vi "BT Example 9 - Queue Synch.vi"() -> ()   [LabVIEW 2021]
uses:
  Support/Nodes/abs_Node/Status.ctl
  System/bt_System.lvclass
  Support/Nodes/Composites/abs_Parallel/Support/Status Calculation.ctl
  Blackboard/Blackboard.lvclass
  Support/Nodes/Decorators/Repeater/Support/Finish On - Type.ctl
  Support/Synch Type 1.ctl
  Blackboard/Blackboard.lvclass/Blackboard.ctl
  Support/Nodes/Leaves/abs_Type Leaf/abs_Type Leaf.lvclass/abs_Type Leaf.ctl
  Blackboard/Get Value Type/Get I32.vi
  Blackboard/Support/Index Group.vi
  Blackboard/Support/Index Tags.vi
  Support/Nodes/Leaves/abs_Type Leaf/Properties/Write Value Class.vi
  <vilib>/TSA/Omni-Bus/Local Bus/Support/I32/Local Bus_I32.lvclass
  C:/Program Files (x86)/National Instruments/LabVIEW 2021/vi.lib/TSA/Abstract Data Classes/Abs_Types/Value/Abs_Value.lvclass
  <vilib>/TSA/Abstract Data Classes/Abs_Types/I32 Integer/Abs_I32 Integer.lvclass
  C:/Program Files (x86)/National Instruments/LabVIEW 2021/vi.lib/TSA/Abstract Data Classes/Abs_Types/Numeric/Abs_Numeric.lvclass
  Support/Nodes/Leaves/Test Boolean/Test Abs_Boolean.lvclass
  C:/Users/Tim/Documents/GitHub/LV_Behaviour_Tree/Source/Support/Nodes/abs_Node/bt_Node.lvclass
  C:/Users/Tim/Documents/GitHub/LV_Behaviour_Tree/Source/Support/Nodes/Leaves/abs_Type Leaf/abs_Type Leaf.lvclass
  <vilib>/TSA/Abstract Data Classes/Abs_Types/Boolean/Abs_Boolean.lvclass
  C:/Program Files (x86)/National Instruments/LabVIEW 2021/vi.lib/TSA/Abstract Data Classes/Abs_Types/Type/Abs_Type.lvclass
  <vilib>/TSA/Omni-Bus/Local Bus/Support/Initialise DVR's.vi
  <vilib>/TSA/Abstract Data Classes/Functions/Math/Support/Increment/I32/Method.vi
  <vilib>/TSA/Abstract Data Classes/Constants/Support/I32/I32.vi
  <vilib>/TSA/Abstract Data Classes/Functions/Compare/Support/Greater Equal/I32/Method.vi
  <vilib>/TSA/Abstract Data Classes/Abs_Types/Value/Abs_Value.lvclass
  <vilib>/TSA/Abstract Data Classes/Abs_Types/Type/Abs_Type.lvclass
  <vilib>/TSA/Omni-Bus/Local Bus/Support/DBL/Local Bus_DBL.lvclass
  <vilib>/TSA/Omni-Bus/Local Bus/Support/SGL/Local Bus_SGL.lvclass
  <vilib>/TSA/Omni-Bus/Local Bus/Support/EXT/Local Bus_EXT.lvclass
  <vilib>/TSA/Omni-Bus/Local Bus/Support/Bool/Local Bus_Boolean.lvclass
  <vilib>/TSA/Omni-Bus/Local Bus/Support/STR/Local Bus_String.lvclass
  <vilib>/TSA/Omni-Bus/Local Bus/Support/Variant/Local Bus_Variant.lvclass
  <vilib>/TSA/Omni-Bus/Local Bus/Support/WFM/Local Bus_Waveform.lvclass
  <vilib>/TSA/Omni-Bus/Local Bus/Support/Time/Local Bus_Time.lvclass
  <vilib>/TSA/Omni-Bus/Local Bus/Support/U8/Local Bus_U8.lvclass
  <vilib>/TSA/Omni-Bus/Local Bus/Support/U16/Local Bus_U16.lvclass
  <vilib>/TSA/Omni-Bus/Local Bus/Support/U32/Local Bus_U32.lvclass
  <vilib>/TSA/Omni-Bus/Local Bus/Support/U64/Local Bus_U64.lvclass
  <vilib>/TSA/Omni-Bus/Local Bus/Support/I8/Local Bus_I8.lvclass
  <vilib>/TSA/Omni-Bus/Local Bus/Support/I16/Local Bus_I16.lvclass
  <vilib>/TSA/Omni-Bus/Local Bus/Support/I64/Local Bus_I64.lvclass
  <vilib>/TSA/Omni-Bus/Local Bus/Support/CSGL/Local Bus_CSGL.lvclass
  <vilib>/TSA/Omni-Bus/Local Bus/Support/CDBL/Local Bus_CDBL.lvclass
  <vilib>/TSA/Omni-Bus/Local Bus/Support/CEXT/Local Bus_CEXT.lvclass
  <vilib>/TSA/Omni-Bus/Local Bus/Support/Type/Local Bus_Type.lvclass
  BT.lvlib
  Support/Nodes/Composites/abs_Parallel/bt_Parallel.lvclass
  Support/Nodes/Decorators/Repeater/bt_Repeater.lvclass
  C:/Program Files (x86)/National Instruments/LabVIEW 2021/vi.lib/TSA/Abstract Data Classes/Abs_Types/Integer/Abs_Integer.lvclass
  C:/Program Files (x86)/National Instruments/LabVIEW 2021/vi.lib/TSA/Abstract Data Classes/Abs_Types/I32 Integer/Abs_I32 Integer.lvclass
  <vilib>/TSA/Abstract Data Classes/Constants/Support/I32/Const_I32.lvclass
  <vilib>/TSA/Abstract Data Classes/Functions/Compare/Support/Greater Equal/I32/Greater Equal_I32.lvclass
  <vilib>/TSA/Abstract Data Classes/Functions/Math/Support/Increment/I32/Increment_I32.lvclass
  Support/Nodes/abs_Node/bt_Node.lvclass
panel:
  out "Tags Table":string[][](table)
  out "error out":errorcluster
  in  "stop":bool
  out "Status":T1
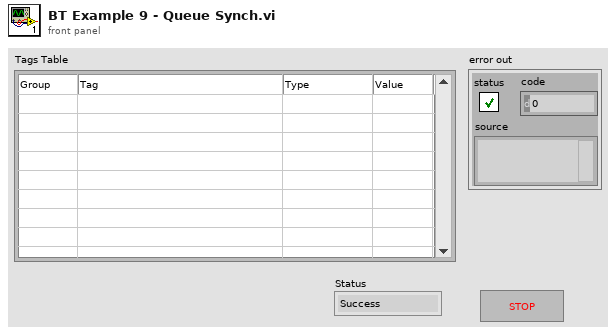
[diagram p1: front panel]
types:
  T1 = typedef "BT.lvlib/bt_Node.lvclass/Status.ctl" = enum16{"Success", "Failure", "Running"}
  T2 = typedef "Synch Type 1.ctl" = cluster{"n":i32, "Bool":bool, "Str":string, "Cluster":cluster{"Numeric":dbl, "Waveform":waveform(dbl), "Time Stamp":timestamp, "Variant":variant}}
  T3 = typedef "BT.lvlib/bt_Repeater.lvclass/Finish On - Type.ctl" = enum16{"Success", "Failure", "Never"}
  T4 = typedef "BT.lvlib/bt_Parallel.lvclass/Status Calculation.ctl" = enum16{"Succeed on All Succeed", "Failure on All Failure", "Succeed on Any Succeed", "Failure on Any Failure"}
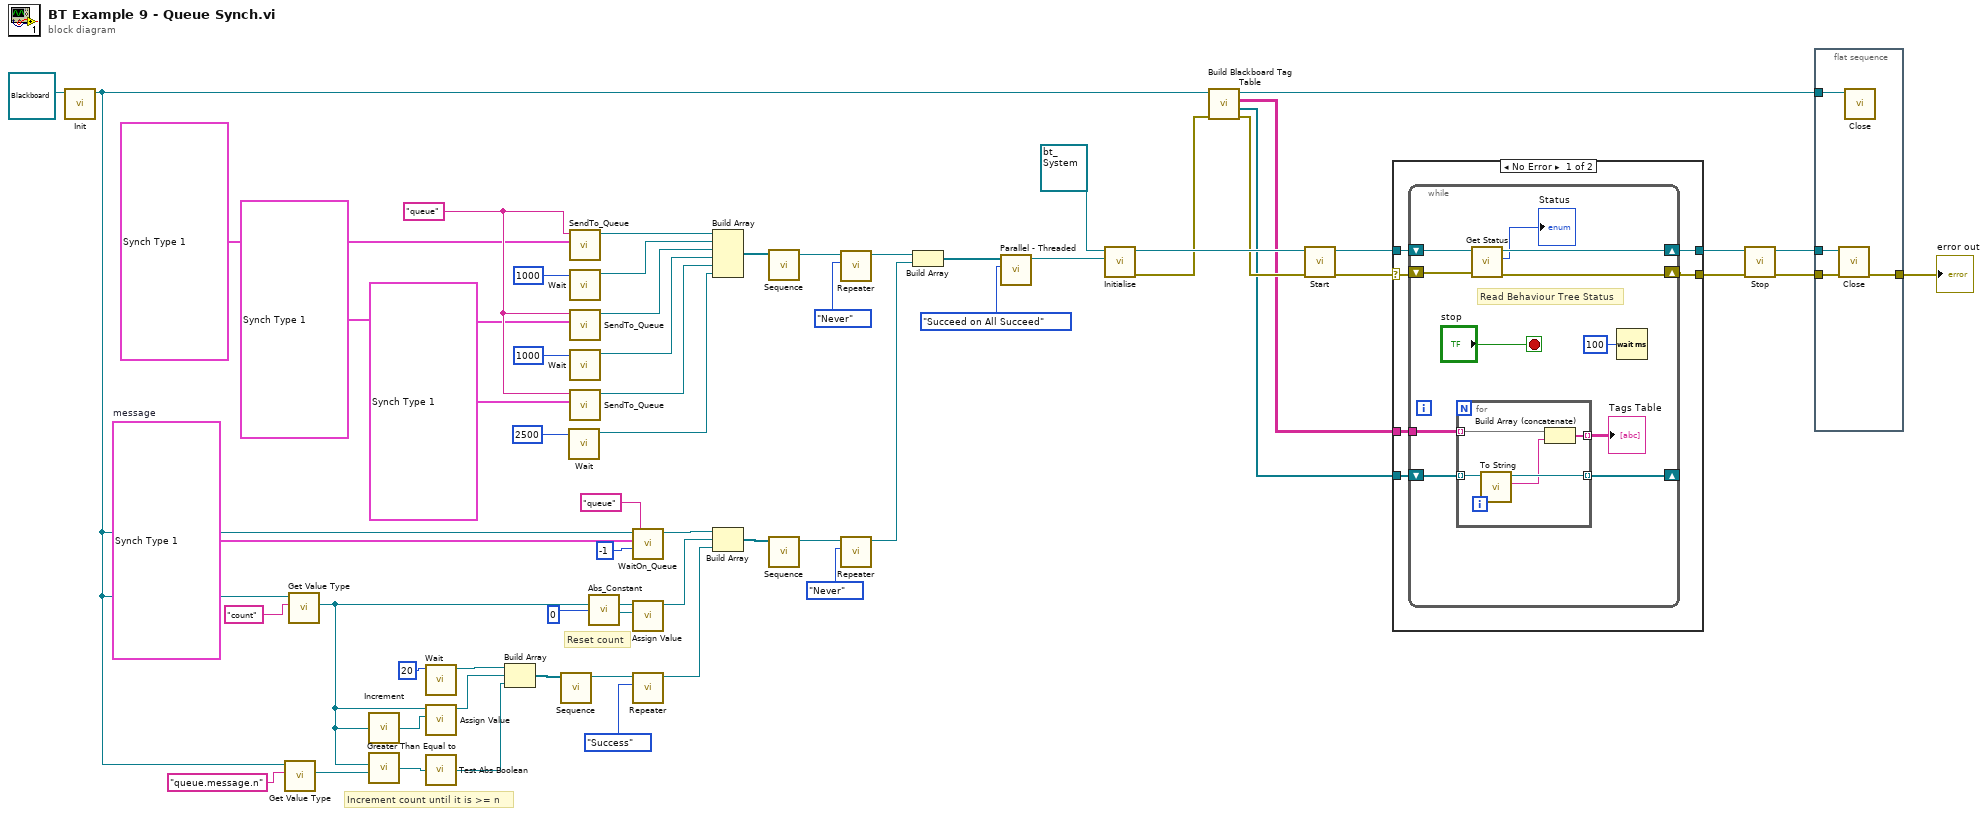
[diagram p0: block diagram]
diagram:
  w4 = T2 {"n"=0, "Bool"=TRUE, "Str"="", "Cluster"={"Numeric"=0.0, "Waveform"={"t0"=timestamp(0 s since 1904-01-01), "dt"=4.0, "Y"=[]}, "Time Stamp"=timestamp(0 s since 1904-01-01), "Variant"=variant}}  # message
  w10 = "queue" ("Name")
  # "Increment count until it is >= n"
  # "Reset count"
  n1 = call-dynamic "Init.vi"("bt_Blackboard in"=refnum<class "Blackboard.lvclass"> refnum) -> ("bt_Blackboard out"=w21:refnum<class "Blackboard.lvclass">)  [unwired: 9 in, 1 out]
  n2 = call-poly "Get Value Type.vi"("Tag"="queue.message.n", "Blackboard in"=w21) -> ("Value"=w22:refnum<class "Abs_I32 Integer.lvclass">)  [unwired: 6 in, 3 out]
  n3 = call-poly "Get Value Type.vi"("Tag"="count", "Blackboard in"=w21) -> ("Value"=w23:refnum<class "Abs_I32 Integer.lvclass">)  [unwired: 6 in, 3 out]
  n4 = call-poly <vilib>:"Increment.vi"("Value"=w23) -> ("Result"=w37:refnum<class "Abs_I32 Integer.lvclass">)  [unwired: 4 in]
  n5 = call-poly <vilib>:"Greater Than Equal to.vi"("Value B"=w22, "Value A"=w23) -> ("Result"=w35:refnum<class "Abs_Boolean.lvclass">)  [unwired: 4 in]
  n6 = call "Wait.vi"("Time (ms)"=u32 20) -> ("Node Out"=w32:refnum<class "bt_Node.lvclass">)  [unwired: 10 in]
  n7 = call "Assign Value.vi"("Assigned Value"=w37, "Value"=w23) -> ("Node Out"=w36:refnum<class "bt_Node.lvclass">)  [unwired: 9 in]
  n8 = call "Test Abs Boolean.vi"("Abs_Boolean.lvclass"=w35) -> ("abs_Node"=w34:refnum<class "bt_Node.lvclass">)  [unwired: 4 in]
  n9 = Build Array(w32, w36, w34) -> (w42:refnum<class "bt_Node.lvclass">[])
  n10 = call "Sequence.vi"("Nodes"=w42) -> ("Node"=w43:refnum<class "bt_Node.lvclass">)  [unwired: 10 in]
  n11 = call "Wait.vi"("Time (ms)"=u32 2500) -> ("Node Out"=w5:refnum<class "bt_Node.lvclass">)  [unwired: 10 in]
  n12 = call "SendTo_Queue.vi"("Message"=T2 {"n"=10, "Bool"=TRUE, "Str"="A", "Cluster"={"Numeric"=0.0, "Waveform"={"t0"=timestamp(0 s since 1904-01-01), "dt"=1.0, "Y"=[]}, "Time Stamp"=timestamp(0 s since 1904-01-01), "Variant"=variant}} ("message"), "Queue Name"=w10) -> ("Node Out"=w18:refnum<class "bt_Node.lvclass">)  [unwired: 9 in]
  n13 = call "Wait.vi"("Time (ms)"=u32 1000) -> ("Node Out"=w13:refnum<class "bt_Node.lvclass">)  [unwired: 10 in]
  n14 = call "SendTo_Queue.vi"("Message"=T2 {"n"=33, "Bool"=FALSE, "Str"="B", "Cluster"={"Numeric"=0.0, "Waveform"={"t0"=timestamp(0 s since 1904-01-01), "dt"=2.0, "Y"=[]}, "Time Stamp"=timestamp(0 s since 1904-01-01), "Variant"=variant}} ("data"), "Queue Name"=w10) -> ("Node Out"=w16:refnum<class "bt_Node.lvclass">)  [unwired: 9 in]
  n15 = call "Wait.vi"("Time (ms)"=u32 1000) -> ("Node Out"=w11:refnum<class "bt_Node.lvclass">)  [unwired: 10 in]
  n16 = call "SendTo_Queue.vi"("Message"=T2 {"n"=100, "Bool"=TRUE, "Str"="C", "Cluster"={"Numeric"=0.0, "Waveform"={"t0"=timestamp(0 s since 1904-01-01), "dt"=3.0, "Y"=[]}, "Time Stamp"=timestamp(0 s since 1904-01-01), "Variant"=variant}} ("data"), "Queue Name"=w10) -> ("Node Out"=w15:refnum<class "bt_Node.lvclass">)  [unwired: 9 in]
  n17 = call-poly <vilib>:"Abs_Constant.vi"("Value"=0 ("n")) -> ("Constant"=w38:refnum<class "Abs_I32 Integer.lvclass">)  [unwired: 4 in]
  n18 = call "WaitOn_Queue.vi"("Queue Name"="queue" ("Name"), "Timeout (ms)"=-1, "Message Type"=w4, "bt_Blackboard in"=w21) -> ("Node Out"=w24:refnum<class "bt_Node.lvclass">)  [unwired: 6 in, 1 out]
  n19 = call "Assign Value.vi"("Assigned Value"=w38, "Value"=w23) -> ("Node Out"=w33:refnum<class "bt_Node.lvclass">)  [unwired: 9 in]
  n20 = call "Repeater.vi"("Finish On"=Finish_On_-_Type."Success", "Node In"=w43) -> ("Node Out"=w44:refnum<class "bt_Node.lvclass">)  [unwired: 9 in]
  n21 = Build Array(w18, w13, w16, w11, w15, w5) -> (w17:refnum<class "bt_Node.lvclass">[])
  n22 = Build Array(w24, w33, w44) -> (w46:refnum<class "bt_Node.lvclass">[])
  n23 = call "Sequence.vi"("Nodes"=w17) -> ("Node"=w8:refnum<class "bt_Node.lvclass">)  [unwired: 10 in]
  n24 = call "Sequence.vi"("Nodes"=w46) -> ("Node"=w45:refnum<class "bt_Node.lvclass">)  [unwired: 10 in]
  n25 = call "Repeater.vi"("Finish On"=Finish_On_-_Type."Never", "Node In"=w8) -> ("Node Out"=w7:refnum<class "bt_Node.lvclass">)  [unwired: 9 in]
  n26 = call "Repeater.vi"("Finish On"=Finish_On_-_Type."Never", "Node In"=w45) -> ("Node Out"=w52:refnum<class "bt_Node.lvclass">)  [unwired: 9 in]
  n27 = Build Array(w7, w52) -> (w55:refnum<class "bt_Node.lvclass">[])
  n28 = call "Parallel - Threaded.vi"("Status Calculation"=Status_Calculation."Succeed on All Succeed", "Nodes"=w55) -> ("Node"=w54:refnum<class "bt_Node.lvclass">)  [unwired: 9 in]
  n29 = call "Initialise.vi"("Behaviour Tree"=w54, "bt_System in"=refnum<class "bt_System.lvclass"> refnum) -> ("error out"=w25:errorcluster, "bt_System out"=w28:refnum<class "bt_System.lvclass">)  [unwired: 8 in]
  n30 = call "Build Blackboard Tag Table.vi"("error in (no error)"=w25, "Blackboard in"=w21) -> ("error out"=w27:errorcluster, "Values"=w20:refnum<class "Abs_Value.lvclass">[], "Table"=w19:string[][], "Blackboard out"=w26:refnum<class "Blackboard.lvclass">)  [unwired: 6 in]
  n31 = call "Start.vi"("error in (no error)"=w27, "bt_System in"=w28) -> ("error out"=w49:errorcluster, "bt_System out"=w60:refnum<class "bt_System.lvclass">)  [unwired: 8 in]
  n32 = case shown="No Error" w49 {
    selector: w49 -> [w65 w84]
    tunnel: w60 -> [w67 w85]
    tunnel: [w66 w85] -> w57
    tunnel: [w64 w84] -> w47
    tunnel: w20 -> [w63 _]
    tunnel: w19 -> [w62 _]
    frame No Error {
      n33 = while {
        shift-right: [w76] -> w66
        shift-left: w67 -> [w77]
        shift-right: [w72] -> w64
        shift-left: w65 -> [w73]
        shift-right: [w71] -> _
        shift-left: w63 -> [w70]
        tunnel: w62 -> [w69]
        stop <- "stop" stop-if-true
        # "Read Behaviour Tree Status"
        n34 = for {
          tunnel: [w83] -> w71 mode=indexing
          tunnel: w70 -> [w82] mode=indexing
          tunnel: w69 -> [w81] mode=indexing
          tunnel: [w79] -> w68 mode=indexing
          n35 = call-dynamic "To String.vi"("Types in"=w82) -> ("String"=w80:string, "Types out"=w83:refnum<class "Abs_Value.lvclass">)  [unwired: 8 in, 1 out]
          n36 = Build Array (concatenate)(w81, w80) -> (w79:string[])
        }
        "Tags Table" <- w68
        n37 = call "Get Status.vi"("error in (no error)"=w73, "bt_System in"=w77) -> ("error out"=w72:errorcluster, "Status"=→"Status":T1, "bt_System out"=w76:refnum<class "bt_System.lvclass">)  [unwired: 7 in]
        n38 = Wait (ms)(milliseconds to wait=u32 100) -> ()  [unwired: 1 out]
      }
    }
    frame Error {
    }
  }
  n39 = call "Stop.vi"("error in (no error)"=w47, "bt_System in"=w57) -> ("error out"=w58:errorcluster, "bt_System out"=w59:refnum<class "bt_System.lvclass">)  [unwired: 8 in]
  n40 = flat-sequence {
    tunnel: w59 -> [w89]
    tunnel: w58 -> [w88]
    tunnel: [w87] -> w48
    tunnel: w26 -> [w86]
    frame #0 {
      n41 = call-dynamic "Close.vi"("error in (no error)"=w88, "bt_System in"=w89) -> ("error out"=w87:errorcluster)  [unwired: 8 in, 1 out]
      n42 = call-dynamic "Close.vi"("bt_Blackboard in"=w86) -> ()  [unwired: 9 in, 2 out]
    }
  }
  "error out" <- w48
